vi "Connection String.vi"(8 "error in (no error)":errorcluster, 11 "SQLite_API in":refnum<class "SQLite_API.lvclass">) -> (0 "error out":errorcluster, 2 "Connected String":string, 3 "SQLite_API out":refnum<class "SQLite_API.lvclass">)   [LabVIEW 2021, in "SQLite_API.lvclass"]
uses:
  <userlib>/John_Lib/DataBase/SQLite_API/SQLite_API.lvclass
  <userlib>/John_Lib/DataBase/SQLite_API/SQLite_API.lvclass/SQLite_API.ctl
  <userlib>/John_Lib/DataBase/DataBase_SQL/DataBase_SQL.lvclass
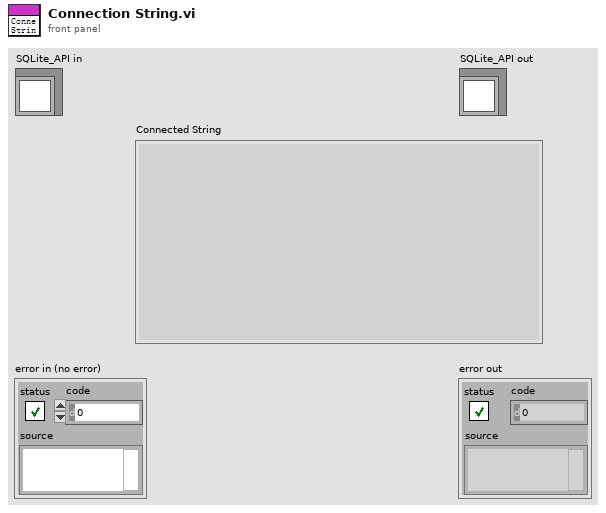
[diagram p1: front panel]
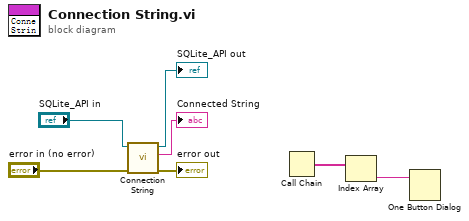
[diagram p0: block diagram]
diagram:
  n1 = call-parent "Connection String.vi"("error in (no error)"="error in (no error)", "DataBase_SQL in"="SQLite_API in") -> ("error out"=→"error out":errorcluster, "Connected String"=→"Connected String":string, "DataBase_SQL out"=→"SQLite_API out":refnum<class "SQLite_API.lvclass">)  [unwired: 7 in]
  n2 = Call Chain() -> (call chain=w2:string[])
  n3 = Index Array(array=w2) -> (element=w1:string)  [unwired: 1 in]
  n4 = One Button Dialog(message=w1) -> ()  [unwired: 1 in, 1 out]
